vi "Configure Trigger.vi"(0 "VISA resource name":refnum<visa-resource-name>, 1 "Trigger Source (0: Immediate)":i32(ring) items=["Immediate", "Timer", "Manual", "Bus", "External"], 5 "Trigger Count (1)":i32=1, 7 "Timer Interval (0.1 s)":dbl=0.1, 9 "Autodelay (T: Enable)":bool=TRUE, 11 "error in (no error)":errorcluster, 12 "Trigger Delay (0 s)":dbl) -> (4 "VISA resource name out":refnum<visa-resource-name>, 15 "error out":errorcluster)   [LabVIEW 2022 SP3, in "Keithley 2182.lvlib"]
doc: "Configures the instrument's trigger layer.\n\n<B>Note:</B>\nThe instrument must be waiting at the control source foe the event when this VI is executed."
uses:
  <instrlib>/Keithley 2182/Keithley 2182.lvlib
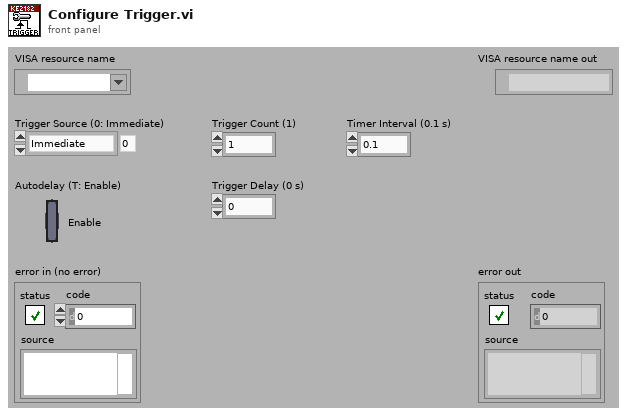
[diagram p1: front panel]
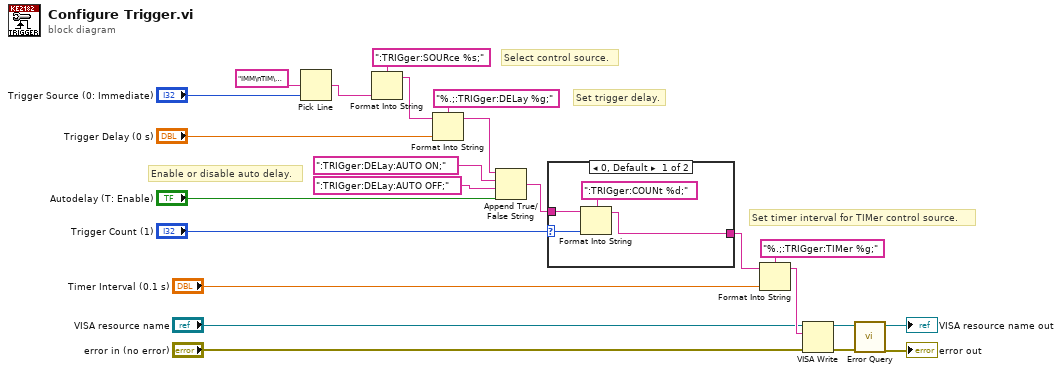
[diagram p0: block diagram]
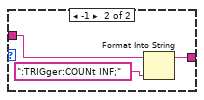
[diagram p2: hidden frame]
diagram:
  # "Set timer interval for TIMer control source."
  # "Enable or disable auto delay."
  # "Set trigger delay."
  # "Select control source."
  n1 = Pick Line(multi-line string="IMM\nTIM\nMAN\nBUS\nEXT", line index="Trigger Source (0: Immediate)") -> (output string=w7:string)  [unwired: 1 in]
  n2 = Format Into String(format string=":TRIGger:SOURce %s;", w7) -> (resulting string=w5:string)  [unwired: 2 in, 1 out]
  n3 = Format Into String(format string="%.;:TRIGger:DELay %g;", initial string=w5, "Trigger Delay (0 s)") -> (resulting string=w4:string)  [unwired: 1 in, 1 out]
  n4 = Append True/False String(1:"Autodelay (T: Enable)", 2:":TRIGger:DELay:AUTO OFF;", 3:":TRIGger:DELay:AUTO ON;", 4:w4) -> (0:w2:string)
  n5 = case shown="0, Default" "Trigger Count (1)" {
    selector: "Trigger Count (1)" -> [w25 _]
    tunnel: w2 -> [w24 w30]
    tunnel: [w26 w28] -> w1
    frame 0, Default {
      n6 = Format Into String(format string=":TRIGger:COUNt %d;", initial string=w24, w25) -> (resulting string=w26:string)  [unwired: 1 in, 1 out]
    }
    frame -1 {
      n7 = Format Into String(initial string=w30, ":TRIGger:COUNt INF;") -> (resulting string=w28:string)  [unwired: 2 in, 1 out]
    }
  }
  n8 = Format Into String(format string="%.;:TRIGger:TIMer %g;", initial string=w1, "Timer Interval (0.1 s)") -> (resulting string=w15:string)  [unwired: 1 in, 1 out]
  n9 = VISA Write(VISA resource name="VISA resource name", write buffer=w15, error in (no error)="error in (no error)") -> (VISA resource name out=w12:refnum<visa-resource-name>, error out=w11:errorcluster)  [unwired: 1 out]
  n10 = call <instrlib>:"Error Query.vi"("error in (no error)"=w11, "VISA resource name"=w12) -> ("error out"=→"error out":errorcluster, "VISA resource name out"=→"VISA resource name out":refnum<visa-resource-name>)  [unwired: 6 in, 2 out]
